vi "Write rotPA.vi"(8 "error in (no error)":errorcluster, 10 "rotPA":dbl[unit] min=0.0 max=6.283185307179586, 11 "Rotator in":refnum<class "Rotator.lvclass">) -> (0 "error out":errorcluster, 3 "Rotator out":refnum<class "Rotator.lvclass">)   [LabVIEW 2022 SP3, in "TCSDataDefinitions.lvlib" / "TCSCommand.lvlib" / "TargetConfiguration.lvlib" / "Rotator.lvclass"]
uses:
  Rotator.lvclass
  Rotator.lvclass/Rotator.ctl
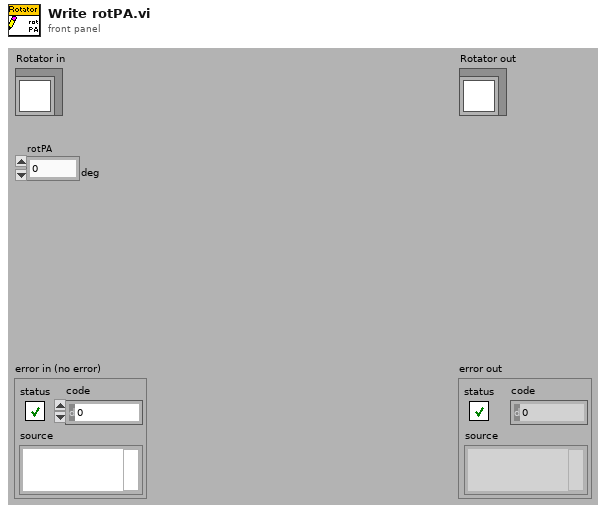
[diagram p1: front panel]
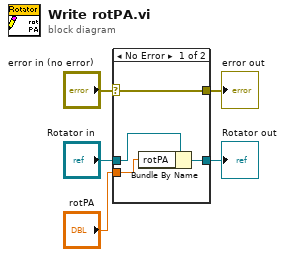
[diagram p0: block diagram]
diagram:
  n1 = case shown="No Error" "error in (no error)" {
    selector: "error in (no error)" -> [w9 w10]
    tunnel: [w9 w10] -> w4
    tunnel: [w7 w11] -> w2
    tunnel: "Rotator in" -> [w8 w11]
    tunnel: "rotPA" -> [w6 _]
    frame No Error {
      n2 = Bundle By Name(cluster=w8, "rotPA"=w6) -> (w7:refnum<class "Rotator.lvclass">)
    }
    frame Error {
    }
  }
  "error out" <- w4
  "Rotator out" <- w2
